vi "Close.vi"(8 "error in":errorcluster, 11 "Cell View in":refnum<class "Cell View.lvclass">) -> (0 "error out":errorcluster, 3 "Cell View out":refnum<class "Cell View.lvclass">)   [LabVIEW 2023, in "SourceGrid.lvlib" / "Cell View.lvclass"]
uses:
  Cell View.lvclass
  Cell View.lvclass/Cell View.ctl
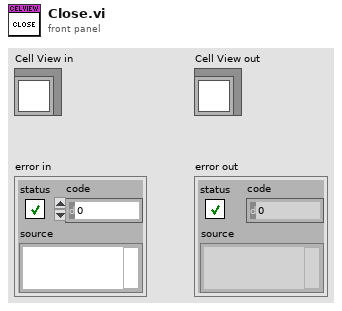
[diagram p1: front panel]
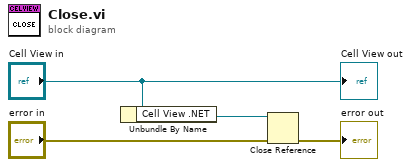
[diagram p0: block diagram]
diagram:
  n1 = Unbundle By Name("Cell View in") -> ("Cell View .NET"=w3:refnum<k24>)
  n2 = Close Reference(reference=w3, error in (no error)="error in") -> (error out=→"error out":errorcluster)
  "Cell View out" <- "Cell View in"
